vi "Stop FGen.vi"(8 "error in (no error)":errorcluster) -> (0 "error out":errorcluster, 3 "queue out":refnum<queue>)   [LabVIEW 2021, in "Queue Library.lvlib"]
uses:
  Queue Library.lvlib
  Controls/Message.ctl
  Controls/State.ctl
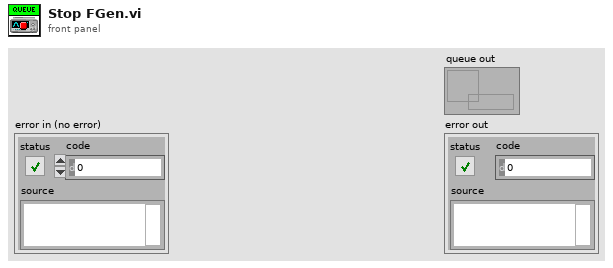
[diagram p1: front panel]
types:
  T1 = typedef "State.ctl" = enum16{"Initialize", "Idle", "Start Scope", "Acquire", "Stop Scope", "Config FGen", "Start FGen", "Sweep FGen", "Stop FGen", "Plot", "Option Selection", "Channel 0 Selection", "Channel 1 Selection", "Update Cursors", "Update Measurements", "Time/Div", "Autoscale", "Stop", "Error"}
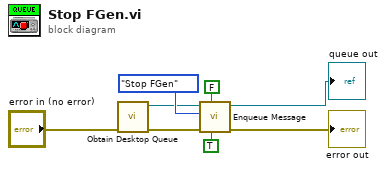
[diagram p0: block diagram]
diagram:
  n1 = call "Obtain Desktop Queue.vi"("error in (no error)"="error in (no error)") -> ("error out"=w6:errorcluster, "queue out"=w5:refnum<queue>)  [unwired: 9 in]
  n2 = call "Enqueue Message.vi"("Priority?"=TRUE, "Flush?"=FALSE, "error in (no error)"=w6, "State"=State."Stop FGen", "queue in"=w5) -> ("error out"=→"error out":errorcluster, "queue out"=→"queue out":refnum<queue>)  [unwired: 5 in]
